vi "Update Plugin Test End Result.vi"(10 "Result":T1, 11 "Execution UI in":refnum<class "Execution UI.lvclass">) -> (3 "Execution UI out":refnum<class "Execution UI.lvclass">)   [LabVIEW 2020, in "Execution UI.lvclass"]
uses:
  Execution UI.lvclass
  Core/Result/Result.ctl
  Core/Result/Status.ctl
  Core/Result/Type.ctl
  Execution UI.lvclass/Execution UI.ctl
  Framework/Plugin/Plugin.lvclass
  Core/Result/Result.lvlib
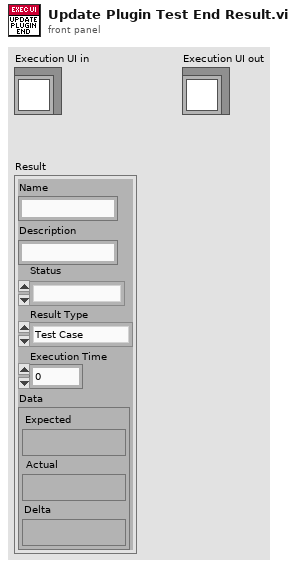
[diagram p1: front panel]
types:
  T1 = typedef "Result.lvlib/Result.ctl" = cluster{"Name":string, "Description":string, "Status":T2, "Result Type":T3, "Execution Time":dbl, "Data":cluster{"Expected":variant, "Actual":variant, "Delta":variant}}
  T2 = typedef "Result.lvlib/Status.ctl" = enum16{"", "Passed", "Failed", "Error", "Skipped", "Setup Error", "Broken", "Teardown Error"}
  T3 = typedef "Result.lvlib/Type.ctl" = enum16{"Test Case", "Test Suite", "Test Run", "Pass", "Fail", "Skip", "Pass if", "Fail if", "Pass if Error", "Fail if Error", "Pass if Equal", "Fail if Equal"}
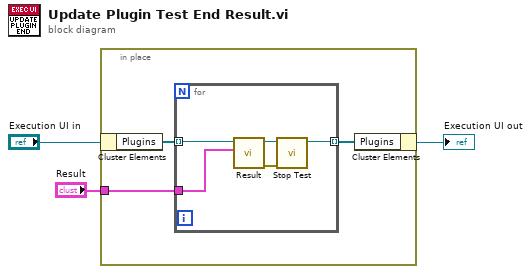
[diagram p0: block diagram]
diagram:
  n1 = in-place {
    in-place-border: "Result" -> [w6]
    n2 = in-place-cluster #1("Execution UI in") -> ("Plugins"=w5:refnum<class "Plugin.lvclass">[])
    n3 = for {
      tunnel: w6 -> [w11]
      tunnel: w5 -> [w9] mode=indexing
      tunnel: [w7] -> w4 mode=indexing
      n4 = call-dynamic "Result.vi"("Result"=w11, "Plugin In"=w9) -> ("error out"=w10:errorcluster, "Plugin Out"=w8:refnum<class "Plugin.lvclass">)  [unwired: 8 in]
      n5 = call-dynamic "Stop Test.vi"("error in (no error)"=w10, "Plugin in"=w8) -> ("Plugin out"=w7:refnum<class "Plugin.lvclass">)  [unwired: 8 in, 1 out]
    }
    n6 = in-place-cluster #1("Plugins"=w4) -> (→"Execution UI out":refnum<class "Execution UI.lvclass">)
  }
